vi "Check If Has Course.vi"(8 "error in (no error)":errorcluster, 10 "CurWeek(0)":i32, 11 "TimeTable in":refnum<class "TimeTable.lvclass">) -> (0 "error out":errorcluster, 2 "Array":string[][](array[string]), 3 "TimeTable out":refnum<class "TimeTable.lvclass">)   [LabVIEW 2015, in "Member_Actor.lvlib" / "TimeTable.lvclass"]
uses:
  TimeTable.lvclass
  TimeTable.lvclass/TimeTable.ctl
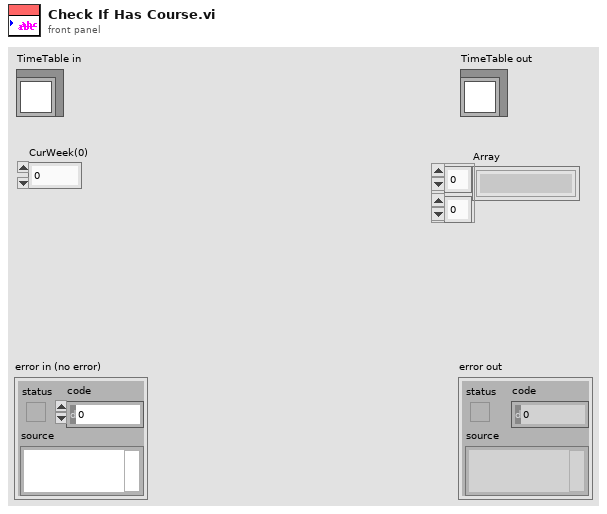
[diagram p1: front panel]
types:
  T1 = typedef "Member_Actor.lvlib/TimeTable.lvclass/Table_Cell.ctl" = cluster{"结束周":i32, "起始周":i32, "课程名称":string}
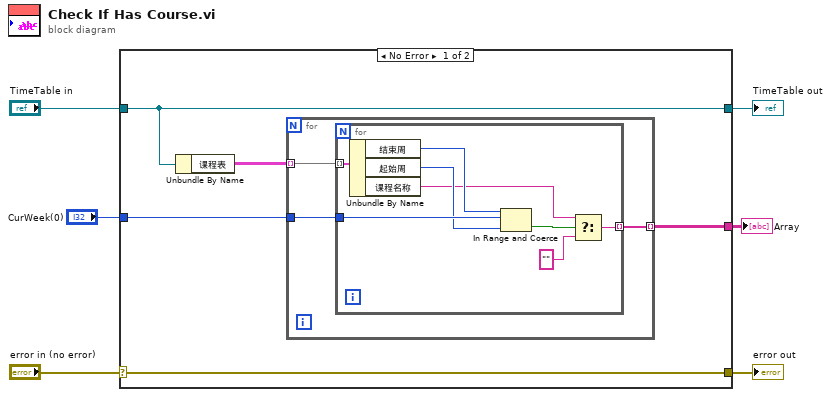
[diagram p0: block diagram]
diagram:
  n1 = case shown="No Error" "error in (no error)" {
    selector: "error in (no error)" -> [w11 w24]
    tunnel: [w11 w24] -> w5
    tunnel: [w10 w23] -> w3
    tunnel: "TimeTable in" -> [w10 w23]
    tunnel: "CurWeek(0)" -> [w8 _]
    tunnel: [w7 _] -> w1
    frame No Error {
      n2 = Unbundle By Name(w10) -> ("课程表"=w9:T1[][])
      n3 = for {
        tunnel: w9 -> [w14] mode=indexing
        tunnel: w8 -> [w13]
        tunnel: [w12] -> w7 mode=indexing
        n4 = for {
          tunnel: w14 -> [w22] mode=indexing
          tunnel: w13 -> [w21]
          tunnel: [w15] -> w12 mode=indexing
          n5 = Unbundle By Name(w22) -> ("结束周"=w20:i32, "起始周"=w19:i32, "课程名称"=w17:string)
          n6 = In Range and Coerce(upper limit=w20, x=w21, lower limit=w19) -> (In Range?=w18:bool)  [unwired: 1 out]
          n7 = Select(t=w17, s=w18, f="") -> (s? t:f=w15:string)
        }
      }
    }
    frame Error {
    }
  }
  "error out" <- w5
  "TimeTable out" <- w3
  "Array" <- w1
